vi "UR Control Command.vi"() -> ()   [LabVIEW 2018]
panel:
  in  "Send String":bool
  in  "Numeric Indicator 2":string
  in  "Numeric Indicator":string
  in  "Command":string="get_target_tcp_pose()"
  in  "Read String":bool
  in  "Get TCP Pose":bool
  in  "Stop":bool
  out "In HEX Format":string
  out "Data Received":string
  out "Error Out":errorcluster
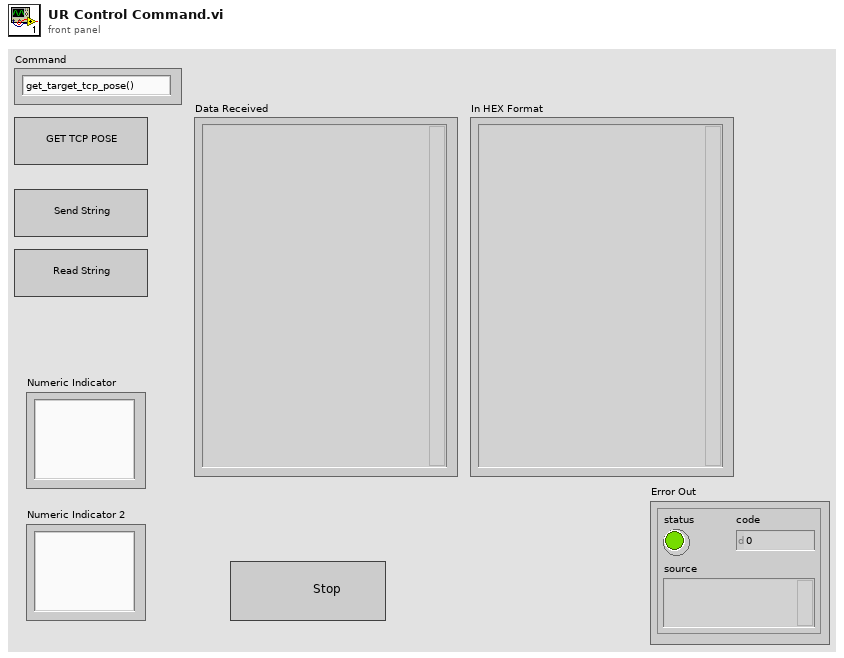
[diagram p1: front panel]
types:
  T1 = enum16{"Standard", "Buffered", "CRLF", "Immediate"}
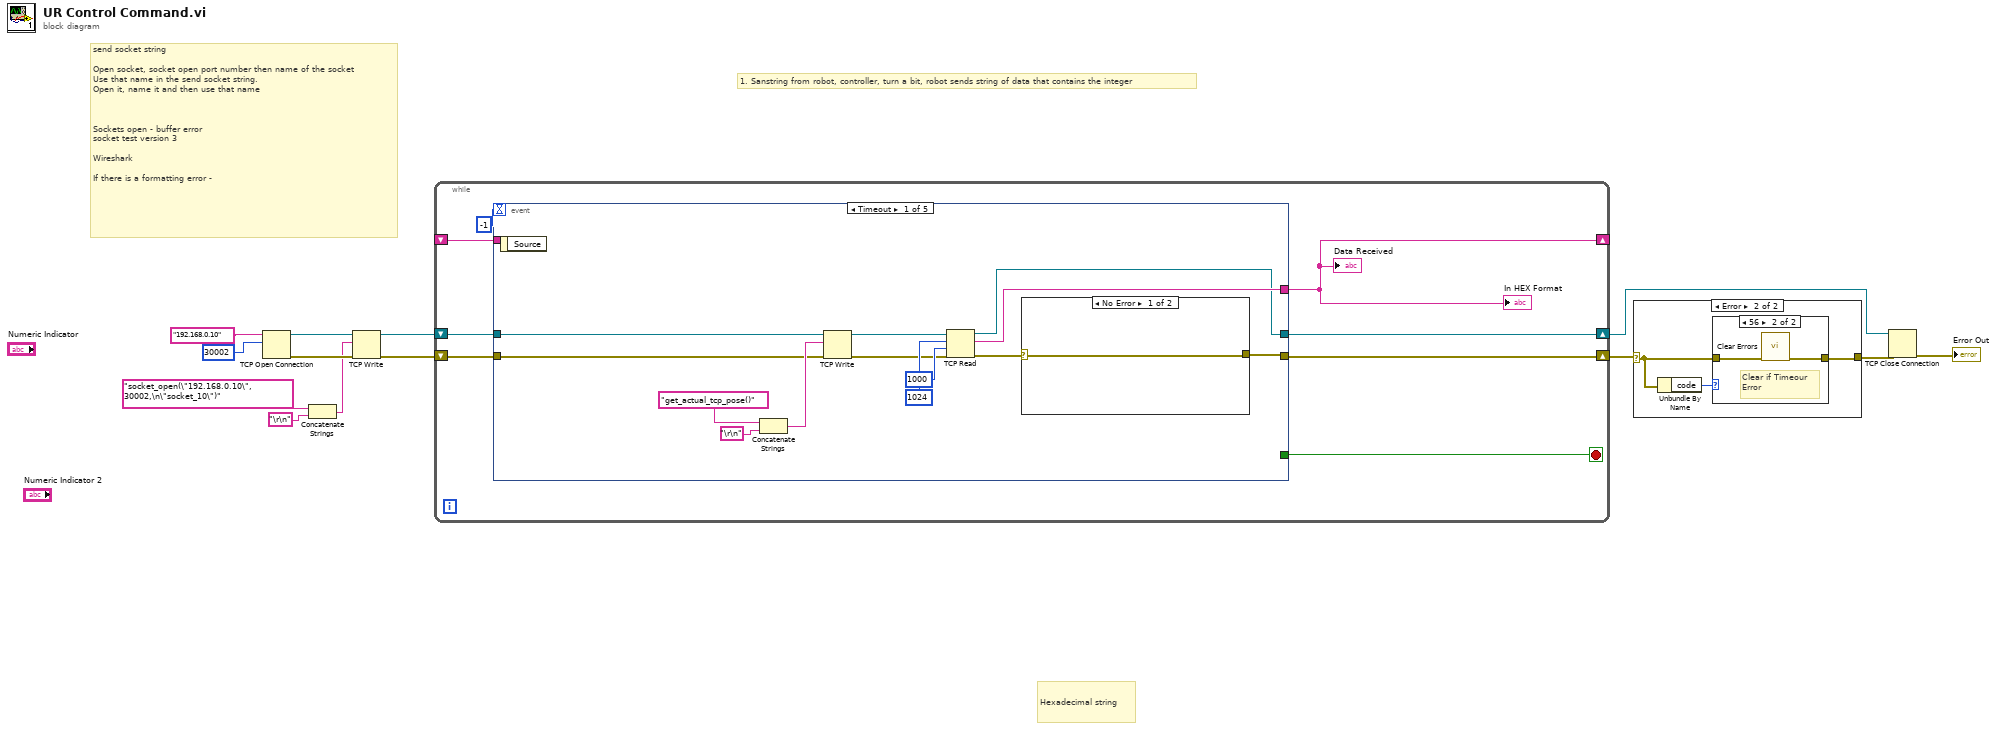
[diagram p0: block diagram]
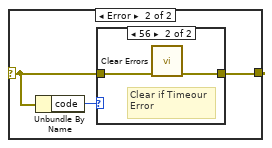
[diagram p2: hidden frame]
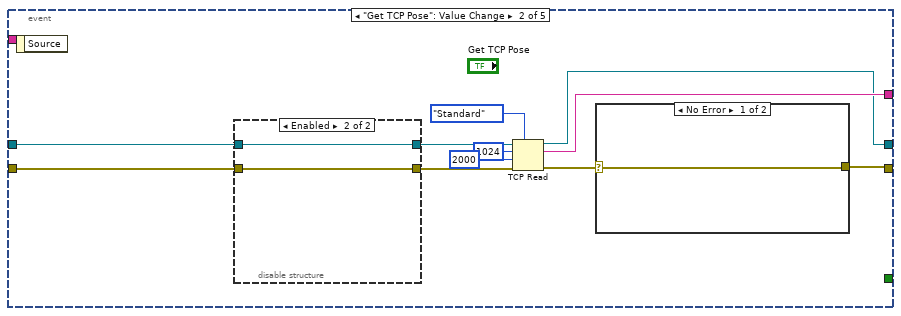
[diagram p4: hidden frame]
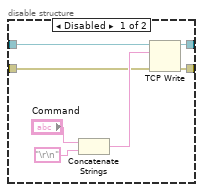
[diagram p5: hidden frame]
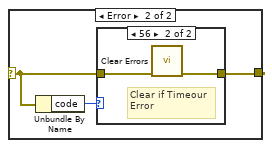
[diagram p6: hidden frame]
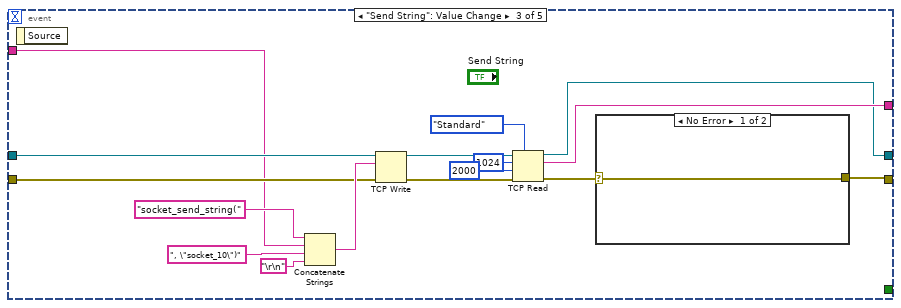
[diagram p8: hidden frame]
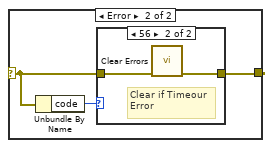
[diagram p9: hidden frame]
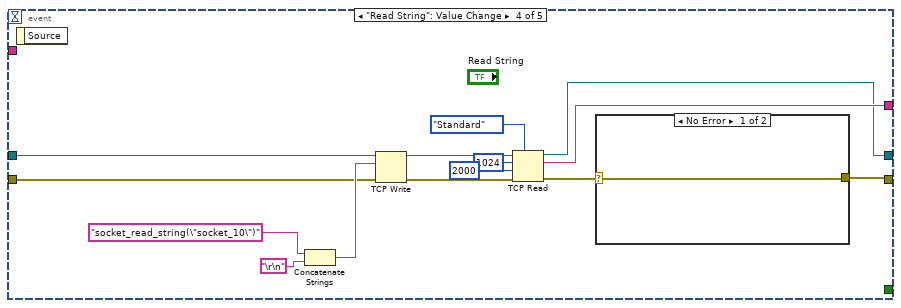
[diagram p11: hidden frame]
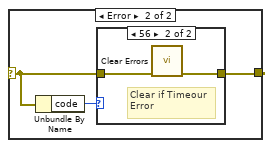
[diagram p12: hidden frame]
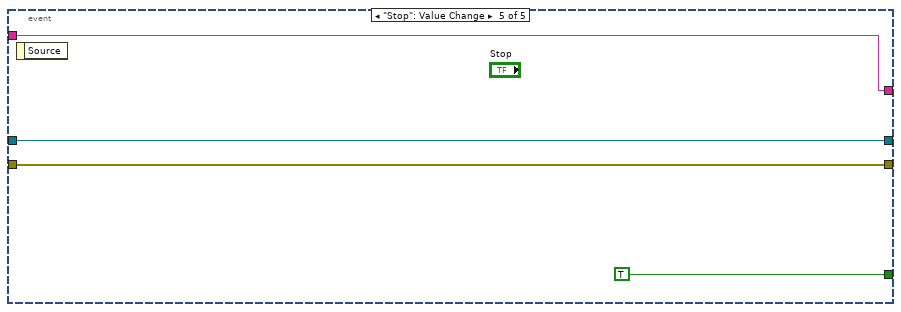
[diagram p14: hidden frame]
diagram:
  # "send socket string\n\nOpen socket, socket open port number then name of the socket\nUse that name in the send socket string.\nOpen it, name it and then use that name\n\n\n\nSockets open - buffer error\nsocket test version 3\n\nWireshark\n\nIf there is a formatting error -"
  # "1. Sanstring from robot, controller, turn a bit, robot sends string of data that contains the integer"
  # "Hexadecimal string"
  n1 = TCP Open Connection(address="192.168.0.10", remote port or service name=u16 30002) -> (connection ID=w5:refnum<k5>, error out=w7:errorcluster)  [unwired: 3 in]
  n2 = Concatenate Strings("socket_open(\"192.168.0.10\", 30002,\n\"socket_10\")" ("string"), "\r\n") -> (w1:string)
  n3 = TCP Write(connection ID=w5, data in=w1, error in (no error)=w7) -> (connection ID out=w4:refnum<k5>, error out=w6:errorcluster)  [unwired: 1 in, 1 out]
  n4 = while {
    shift-right: [w19] -> w8
    shift-left: w4 -> [w20]
    shift-right: [w17] -> w10
    shift-left: w6 -> [w18]
    shift-right: [w14] -> _
    shift-left: _ -> [w15]
    stop <- w21 stop-if-true
    n5 = event shown="[0] Timeout" {
      selector: _ -> [_ _ _ _ _]
      dyn-events: _ -> [_ _ _ _ _]
      timeout: -1 -> [_ _ _ _ _]
      tunnel: [_ _ _ _ TRUE] -> w21
      tunnel: w20 -> [w27 w49 w79 w100 w115]
      tunnel: [w22 w44 w74 w95 w115] -> w19
      tunnel: [w24 w46 w76 w97 w114] -> w17
      tunnel: w18 -> [w26 w48 w78 w99 w114]
      tunnel: [w23 w45 w75 w96 w113] -> w14
      tunnel: w15 -> [_ _ w69 _ w113]
      event Timeout {
        n6 = event-data() -> ()  [unwired: 1 in, 1 out]
        n7 = Concatenate Strings("get_actual_tcp_pose()" ("string"), "\r\n") -> (w32:string)
        n8 = TCP Write(connection ID=w27, data in=w32, error in (no error)=w26) -> (connection ID out=w34:refnum<k5>, error out=w25:errorcluster)  [unwired: 1 in, 1 out]
        n9 = TCP Read(connection ID=w34, bytes to read=1024, error in (no error)=w25, 9:1000 ("timeout ms (25000)")) -> (connection ID out=w22:refnum<k5>, data out=w23:string, error out=w33:errorcluster)  [unwired: 1 in]
        n10 = case shown="No Error" w33 {
          selector: w33 -> [w35 w37]
          tunnel: [w35 w36] -> w24
          frame No Error {
          }
          frame Error {
            n11 = Unbundle By Name(w37) -> ("code"=w38:i32)
            n12 = case shown="56" w38 {
              tunnel: w37 -> [w39 w41]
              tunnel: [w39 w40] -> w36
              frame 0, Default {
              }
              frame 56 {
                # "Clear if Timeour\nError"
                n13 = call <vilib>:"Clear Errors.vi"("error in (no error)"=w41) -> ("error out"=w40:errorcluster)  [unwired: 5 in, 1 out]
              }
            }
          }
        }
      }
      event "Get TCP Pose": Value Change {
        n14 = event-data() -> ()  [unwired: 1 in, 1 out]
        n15 = disable-structure shown="Enabled" {
          disable-tunnel: [w59 w61] -> w52
          disable-tunnel: w49 -> [w55 w61]
          disable-tunnel: w48 -> [w54 w60]
          disable-tunnel: [w53 w60] -> w47
          frame Disabled {
            n16 = Concatenate Strings("Command", "\r\n") -> (w58:string)
            n17 = TCP Write(connection ID=w55, data in=w58, error in (no error)=w54) -> (connection ID out=w59:refnum<k5>, error out=w53:errorcluster)  [unwired: 1 in, 1 out]
          }
          frame Enabled {
          }
        }
        n18 = TCP Read(connection ID=w52, bytes to read=1024, error in (no error)=w47, 7:T1."Standard" ("mode (standard)"), 9:2000 ("timeout ms (25000)")) -> (connection ID out=w44:refnum<k5>, data out=w45:string, error out=w51:errorcluster)
        n19 = case shown="No Error" w51 {
          selector: w51 -> [w62 w64]
          tunnel: [w62 w63] -> w46
          frame No Error {
          }
          frame Error {
            n20 = Unbundle By Name(w64) -> ("code"=w65:i32)
            n21 = case shown="56" w65 {
              tunnel: w64 -> [w66 w68]
              tunnel: [w66 w67] -> w63
              frame 0, Default {
              }
              frame 56 {
                # "Clear if Timeour\nError"
                n22 = call <vilib>:"Clear Errors.vi"("error in (no error)"=w68) -> ("error out"=w67:errorcluster)  [unwired: 5 in, 1 out]
              }
            }
          }
        }
      }
      event "Send String": Value Change {
        n23 = event-data() -> ()  [unwired: 1 in, 1 out]
        n24 = Concatenate Strings("socket_send_string(", w69, ", \"socket_10\")", "\r\n") -> (w82:string)
        n25 = TCP Write(connection ID=w79, data in=w82, error in (no error)=w78) -> (connection ID out=w84:refnum<k5>, error out=w77:errorcluster)  [unwired: 1 in, 1 out]
        n26 = TCP Read(connection ID=w84, bytes to read=1024, error in (no error)=w77, 7:T1."Standard" ("mode (standard)"), 9:2000 ("timeout ms (25000)")) -> (connection ID out=w74:refnum<k5>, data out=w75:string, error out=w83:errorcluster)
        n27 = case shown="No Error" w83 {
          selector: w83 -> [w85 w87]
          tunnel: [w85 w86] -> w76
          frame No Error {
          }
          frame Error {
            n28 = Unbundle By Name(w87) -> ("code"=w88:i32)
            n29 = case shown="56" w88 {
              tunnel: w87 -> [w89 w91]
              tunnel: [w89 w90] -> w86
              frame 0, Default {
              }
              frame 56 {
                # "Clear if Timeour\nError"
                n30 = call <vilib>:"Clear Errors.vi"("error in (no error)"=w91) -> ("error out"=w90:errorcluster)  [unwired: 5 in, 1 out]
              }
            }
          }
        }
      }
      event "Read String": Value Change {
        n31 = event-data() -> ()  [unwired: 1 in, 1 out]
        n32 = Concatenate Strings("socket_read_string(\"socket_10\")", "\r\n") -> (w103:string)
        n33 = TCP Write(connection ID=w100, data in=w103, error in (no error)=w99) -> (connection ID out=w105:refnum<k5>, error out=w98:errorcluster)  [unwired: 1 in, 1 out]
        n34 = TCP Read(connection ID=w105, bytes to read=1024, error in (no error)=w98, 7:T1."Standard" ("mode (standard)"), 9:2000 ("timeout ms (25000)")) -> (connection ID out=w95:refnum<k5>, data out=w96:string, error out=w104:errorcluster)
        n35 = case shown="No Error" w104 {
          selector: w104 -> [w106 w108]
          tunnel: [w106 w107] -> w97
          frame No Error {
          }
          frame Error {
            n36 = Unbundle By Name(w108) -> ("code"=w109:i32)
            n37 = case shown="56" w109 {
              tunnel: w108 -> [w110 w112]
              tunnel: [w110 w111] -> w107
              frame 0, Default {
              }
              frame 56 {
                # "Clear if Timeour\nError"
                n38 = call <vilib>:"Clear Errors.vi"("error in (no error)"=w112) -> ("error out"=w111:errorcluster)  [unwired: 5 in, 1 out]
              }
            }
          }
        }
      }
      event "Stop": Value Change {
        n39 = event-data() -> ()  [unwired: 1 in, 1 out]
      }
    }
    "In HEX Format" <- w14
    "Data Received" <- w14
  }
  n40 = case shown="Error" w10 {
    selector: w10 -> [w117 w119]
    tunnel: [w117 w118] -> w9
    frame No Error {
    }
    frame Error {
      n41 = Unbundle By Name(w119) -> ("code"=w120:i32)
      n42 = case shown="56" w120 {
        tunnel: w119 -> [w121 w123]
        tunnel: [w121 w122] -> w118
        frame 0, Default {
        }
        frame 56 {
          # "Clear if Timeour\nError"
          n43 = call <vilib>:"Clear Errors.vi"("error in (no error)"=w123) -> ("error out"=w122:errorcluster)  [unwired: 5 in, 1 out]
        }
      }
    }
  }
  n44 = TCP Close Connection(connection ID=w8, error in (no error)=w9) -> (error out=→"Error Out":errorcluster)  [unwired: 1 in, 1 out]
